vi "TDMS Mode Channel Page.vi"(8 "error in (no error)":errorcluster, 11 "Node Ptr":T2 format="%.0x") -> (0 "error out":errorcluster)   [LabVIEW 2011, in "TDMS Custom Device.lvlib"]
uses:
  TDMS Custom Device.lvlib
  <vilib>/NI Veristand/Custom Device API/Custom Device Item Ref.ctl
  <vilib>/NI Veristand/Custom Device API/Custom Device API.lvlib
panel:
  in  "Initial mode":T1(ring)=enum."Loop"
  in  "Header":cluster{"Section Name":string}={"Section Name"="TDMS Mode Channel Settings"}
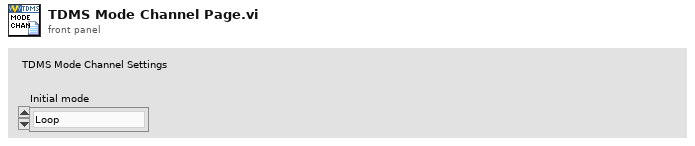
[diagram p1: front panel]
types:
  T1 = enum16{"Play and Repeat Last", "Stop (and Reset)", "Loop", "Pause"}
  T2 = typedef "Custom Device API.lvlib/Custom Device Item Ref.ctl" = u64
  T3 = typedef "Custom Device API.lvlib/Custom Device Channel.ctl" = cluster{"Type":T4, "Units":string, "Default Value":dbl, "Faultable":bool, "Scalable":bool}
  T4 = typedef "Custom Device API.lvlib/Custom Device Channel Type.ctl" = enum16{"Input", "Output"}
  T5 = typedef "Custom Device API.lvlib/Custom Device Commands.ctl" = enum16{"Default", "Item renamed", "Shutdown", "Dynamic button pressed"}
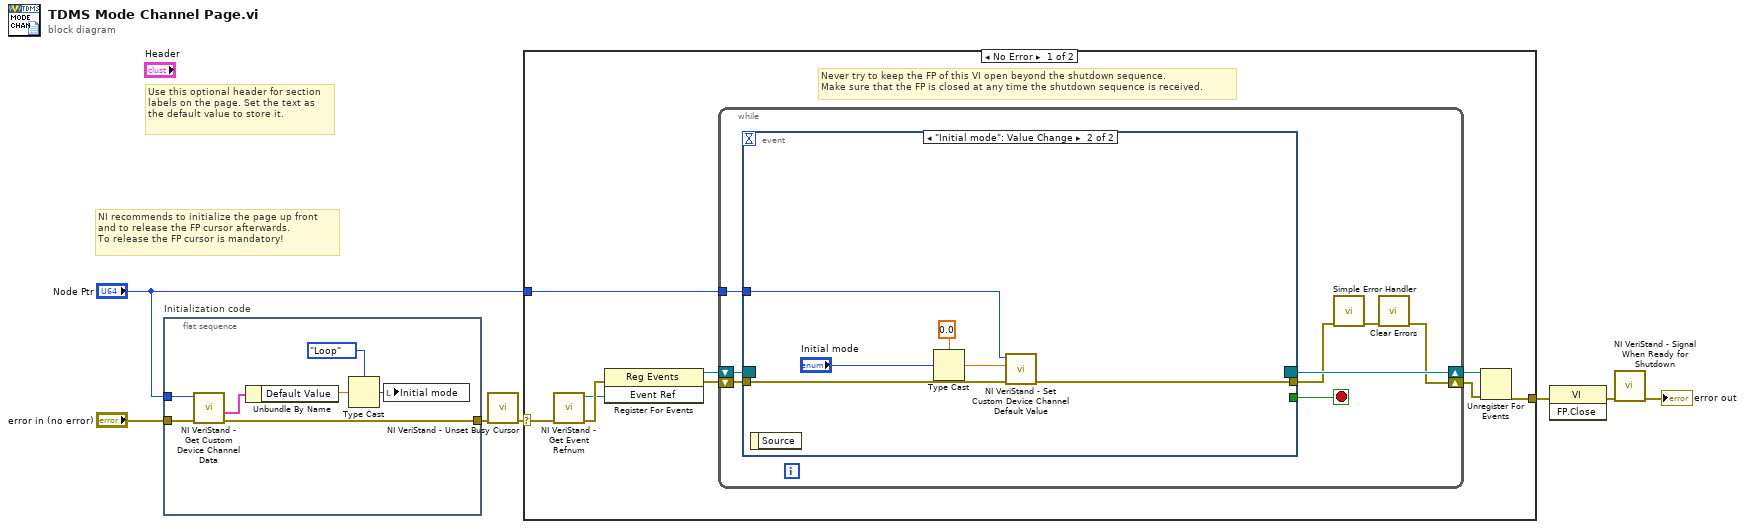
[diagram p0: block diagram]
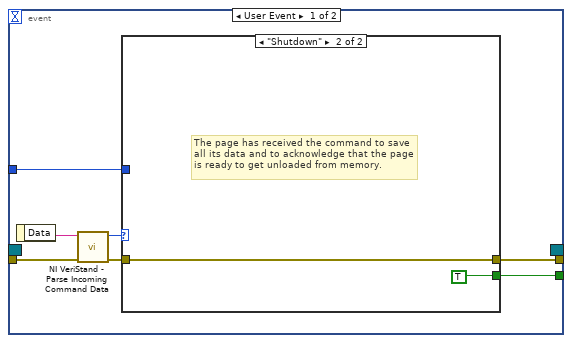
[diagram p2: hidden frame]
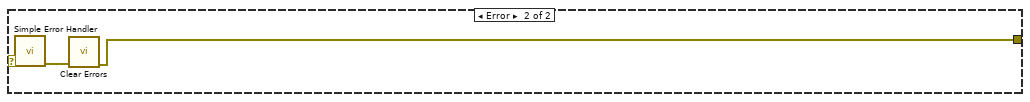
[diagram p4: hidden frame]
diagram:
  # "Use this optional header for section labels on the page. Set the text as the default value to store it."
  # "NI recommends to initialize the page up front\nand to release the FP cursor afterwards.\nTo release the FP cursor is mandatory!"
  n1 = flat-sequence "Initialization code" {
    tunnel: "error in (no error)" -> [w10]
    tunnel: "Node Ptr" -> [w9]
    tunnel: [w8] -> w1
    frame #0 {
      n2 = call <vilib>:"NI VeriStand - Get Custom Device Channel Data.vi"("error in (no error)"=w10, "Channel Ref in"=w9) -> ("error out"=w8:errorcluster, "Channel"=w14:T3)  [unwired: 8 out]
      n3 = Unbundle By Name(w14) -> ("Default Value"=w12:dbl)
      n4 = Type Cast(type=T1."Loop" ("Starting mode"), x=w12) -> (*(type *) &x=w13:T1)
      n5 = local write "Initial mode"(w13) -> ()
    }
  }
  n6 = call <vilib>:"NI VeriStand - Unset Busy Cursor.vi"("error in (no error)"=w1) -> ("error out"=w3:errorcluster)  [unwired: 10 out]
  n7 = case shown="No Error" w3 {
    selector: w3 -> [w15 w50]
    tunnel: [w20 w48] -> w7
    tunnel: "Node Ptr" -> [w16 _]
    frame No Error {
      # "Never try to keep the FP of this VI open beyond the shutdown sequence.\nMake sure that the FP is closed at any time the shutdown sequence is received."
      n8 = call <vilib>:"NI VeriStand - Get Event Refnum.vi"("error in (no error)"=w15) -> ("error out"=w23:errorcluster, "Event Ref"=w19:refnum<user-event>)  [unwired: 9 out]
      n9 = register-events(error in=w23, w19) -> (reference out=w17:refnum<event-registration>, error out=w18:errorcluster)  [unwired: 1 in]
      n10 = while {
        tunnel: w16 -> [w27]
        shift-right: [w24] -> w21
        shift-left: w18 -> [w30]
        shift-right: [w31] -> w22
        shift-left: w17 -> [w29]
        stop <- w28 stop-if-true
        n11 = event shown="[1] \"Initial mode\": Value Change" {
          selector: w29 -> [_ _]
          dyn-events: [_ _] -> w31
          timeout: _ -> [_ _]
          tunnel: w30 -> [w38 w46]
          tunnel: [w34 _] -> w28
          tunnel: [w33 w47] -> w26
          tunnel: w27 -> [w32 w45]
          event User Event {
            n12 = event-data() -> ("Data"=w37:string)  [unwired: 1 out]
            n13 = call <vilib>:"NI VeriStand - Parse Incoming Command Data.vi"("error in (no error)"=w38, "Incoming data"=w37) -> ("error out"=w36:errorcluster, "Action"=w35:T5)  [unwired: 8 out]
            n14 = case shown="\"Shutdown\"" w35 {
              tunnel: w36 -> [w39 w40]
              tunnel: [_ TRUE] -> w34
              tunnel: [w39 w40] -> w33
              tunnel: w32 -> [_ _]
              frame "Default", Default {
              }
              frame "Shutdown" {
                # "The page has received the command to save all its data and to acknowledge that the page is ready to get unloaded from memory."
              }
            }
          }
          event "Initial mode": Value Change {
            n15 = event-data() -> ()  [unwired: 2 out]
            n16 = Type Cast(type=0.0, x="Initial mode") -> (*(type *) &x=w43:dbl)
            n17 = call <vilib>:"NI VeriStand - Set Custom Device Channel Default Value.vi"("error in (no error)"=w46, "Default Value"=w43, "Channel Ref in"=w45) -> ("error out"=w47:errorcluster)  [unwired: 8 out]
          }
        }
        n18 = call <vilib>:"Simple Error Handler.vi"("error in (no error)"=w26) -> ("error out"=w25:errorcluster)  [unwired: 1 in, 7 out]
        n19 = call <vilib>:"Clear Errors.vi"("error in (no error)"=w25) -> ("error out"=w24:errorcluster)  [unwired: 6 out]
      }
      n20 = Unregister For Events(event registration refnum=w22, error in=w21) -> (error out=w20:errorcluster)
    }
    frame Error {
      n21 = call <vilib>:"Simple Error Handler.vi"("error in (no error)"=w50) -> ("error out"=w49:errorcluster)  [unwired: 1 in, 7 out]
      n22 = call <vilib>:"Clear Errors.vi"("error in (no error)"=w49) -> ("error out"=w48:errorcluster)  [unwired: 6 out]
    }
  }
  n23 = invoke class="VI" method="FP.Close"(error in=w7) -> (error out=w6:errorcluster)  [unwired: 2 in, 2 out]
  n24 = call <vilib>:"NI VeriStand - Signal When Ready for Shutdown.vi"("error in (no error)"=w6) -> ("error out"=→"error out":errorcluster)  [unwired: 10 out]
